vi "Launcher.vi"() -> (0 "error out":errorcluster)   [LabVIEW 2015]
uses:
  <vilib>/ErrorRing/Error Ring.xnode
  Libraries/Model/Model.lvlib
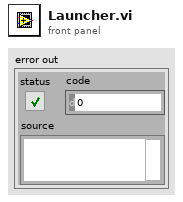
[diagram p1: front panel]
types:
  T1 = cluster{"Minimum Splash Screen Time (ms)":u32, "Splash Screen Start Time (ms)":u32}
  T2 = enum32{"Invalid", "Standard", "Closed", "Hidden", "Minimized", "Maximized"}
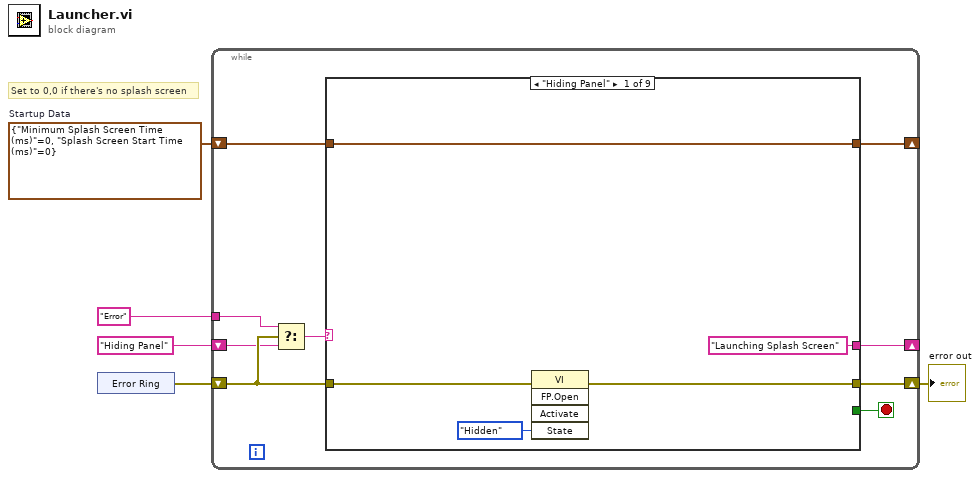
[diagram p0: block diagram]
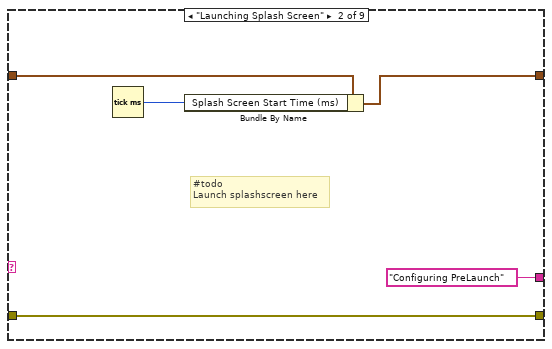
[diagram p2: hidden frame]
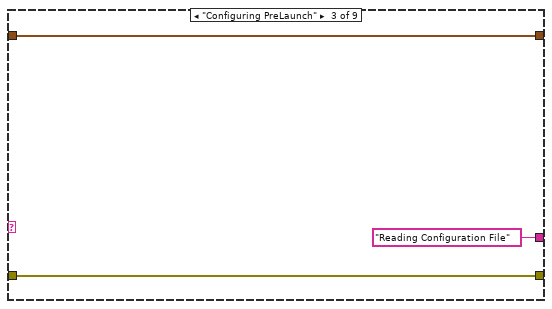
[diagram p3: hidden frame]
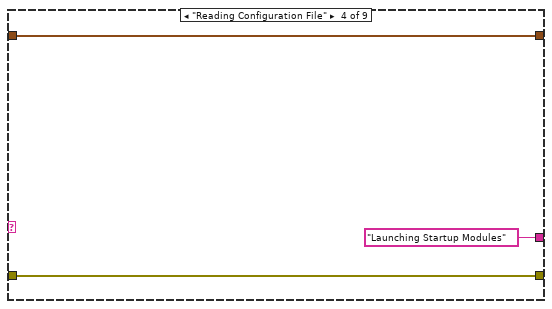
[diagram p4: hidden frame]
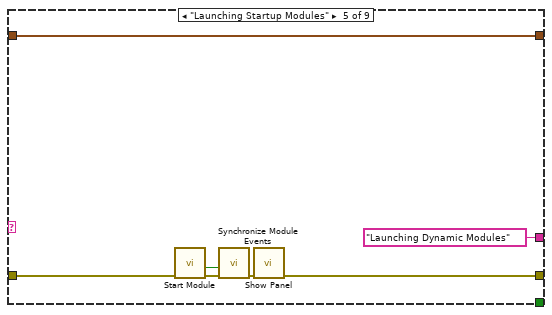
[diagram p5: hidden frame]
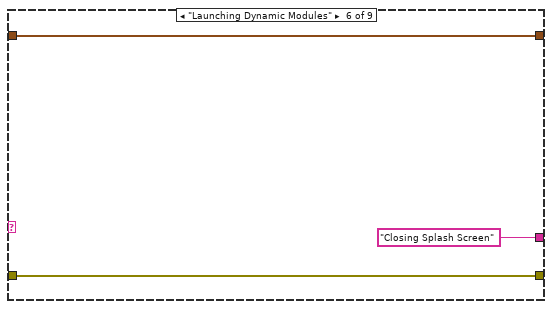
[diagram p6: hidden frame]
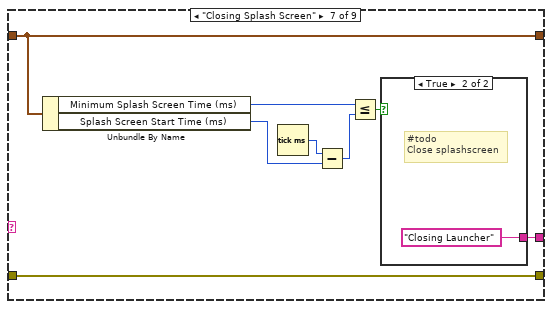
[diagram p7: hidden frame]
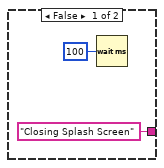
[diagram p8: hidden frame]
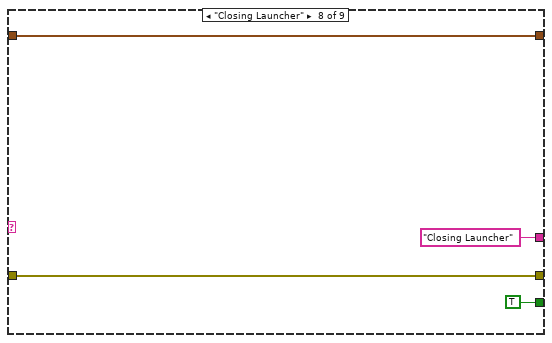
[diagram p9: hidden frame]
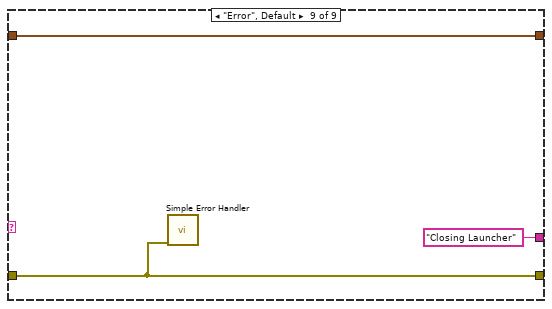
[diagram p10: hidden frame]
diagram:
  w4 = T1 {"Minimum Splash Screen Time (ms)"=0, "Splash Screen Start Time (ms)"=0}  # Startup Data
  # "Set to 0,0 if there's no splash screen"
  n1 = xnode "Error Ring"() -> ("error out"=w3:errorcluster)
  n2 = while {
    shift-right: [w7] -> _
    shift-left: "Hiding Panel" -> [w11]
    shift-right: [w13] -> _
    shift-left: w4 -> [w14]
    shift-right: [w8] -> w1
    shift-left: w3 -> [w12]
    tunnel: "Error" -> [w10]
    stop <- w6 stop-if-true
    n3 = Select(t=w10, s=w12, f=w11) -> (s? t:f=w9:string)
    n4 = case shown="\"Hiding Panel\"" w9 {
      tunnel: w14 -> [w19 w22 w27 w30 w37 w40 w47 w55 w58]
      tunnel: [w19 w20 w27 w30 w37 w40 w47 w55 w58] -> w13
      tunnel: w12 -> [w16 w24 w26 w29 w35 w39 w48 w53 w57]
      tunnel: [w15 w24 w26 w29 w31 w39 w48 w53 w57] -> w8
      tunnel: ["Launching Splash Screen" "Configuring PreLaunch" "Reading Configuration File" "Launching Startup Modules" "Launching Dynamic Modules" "Closing Splash Screen" w41 "Closing Launcher" "Closing Launcher"] -> w7
      tunnel: [_ _ _ _ _ _ _ TRUE _] -> w6
      frame "Hiding Panel" {
        n5 = invoke class="VI" method="FP.Open"(error in=w16, "State"=T2."Hidden") -> (error out=w15:errorcluster)  [unwired: 3 in, 4 out]
      }
      frame "Launching Splash Screen" {
        # "#todo\nLaunch splashscreen here"
        n6 = Tick Count (ms)() -> (millisecond timer value=w21:u32)
        n7 = Bundle By Name(cluster=w22, "Splash Screen Start Time (ms)"=w21) -> (w20:T1)
      }
      frame "Configuring PreLaunch" {
      }
      frame "Reading Configuration File" {
      }
      frame "Launching Startup Modules" {
        n8 = call "Start Module.vi"("error in (no error)"=w35) -> ("error out"=w34:errorcluster, "Wait for Event Sync?"=w33:bool)  [unwired: 7 in, 2 out]
        n9 = call "Synchronize Module Events.vi"("error in (no error)"=w34, "Wait for Event Sync?"=w33) -> ("error out"=w32:errorcluster)  [unwired: 9 in]
        n10 = call "Show Panel.vi"("error in (no error)"=w32) -> ("error out"=w31:errorcluster)  [unwired: 10 in]
      }
      frame "Launching Dynamic Modules" {
      }
      frame "Closing Splash Screen" {
        n11 = Unbundle By Name(w47) -> ("Minimum Splash Screen Time (ms)"=w44:u32, "Splash Screen Start Time (ms)"=w45:u32)
        n12 = Tick Count (ms)() -> (millisecond timer value=w46:u32)
        n13 = Subtract(x=w46, y=w45) -> (x-y=w43:u32)
        n14 = Less Or Equal?(x=w44, y=w43) -> (x <= y?=w42:bool)
        n15 = case shown="True" w42 {
          tunnel: ["Closing Splash Screen" "Closing Launcher"] -> w41
          frame False {
            n16 = Wait (ms)(milliseconds to wait=u32 100) -> ()  [unwired: 1 out]
          }
          frame True {
            # "#todo\nClose splashscreen"
          }
        }
      }
      frame "Closing Launcher" {
      }
      frame "Error", Default {
        n17 = call <vilib>:"Simple Error Handler.vi"("error in (no error)"=w57) -> ()  [unwired: 4 in, 5 out]
      }
    }
  }
  "error out" <- w1
